vi "Actor Core.vi"(8 "error in":errorcluster, 11 "Nested in":refnum<class "Baratron.lvclass">) -> (0 "error out":errorcluster, 3 "Actor out":refnum<class "Actor.lvclass">)   [LabVIEW 2021, in "Baratron.lvclass"]
doc: "(<B>Filename</B>: Actor Framework.lvlib:Actor.lvclass:Actor Core.vi)\n\nReceives messages to the actor, reacts to them, and initiates any error handling that may shut the actor down.\n\nDescendant classes may override this VI to append parallel tasks for the actor to complete while it handles messages. Overrides use the Call Parent Method node."
uses:
  Baratron.lvclass
  C:/Program Files/National Instruments/LabVIEW 2021/vi.lib/ActorFramework/Actor/Actor.lvclass
  <vilib>/ActorFramework/Actor/Actor.lvclass
  Baratron.lvclass/Baratron.ctl
  <vilib>/ActorFramework/Actor/Actor.lvclass/Actor.ctl
  <vilib>/ActorFramework/Message Enqueuer/Message Enqueuer.lvclass/Message Enqueuer.ctl
  <vilib>/ActorFramework/Message Enqueuer/Init from Existing Queue.vi
  <vilib>/ActorFramework/Message Enqueuer/Enqueue.vi
  <vilib>/ActorFramework/Stop Msg/Stop Msg.lvclass
  C:/Program Files/National Instruments/LabVIEW 2021/vi.lib/ActorFramework/Message/Message.lvclass
  <vilib>/ActorFramework/Message Priority Queue/Priority Enqueue.vi
  <vilib>/MGI/Panel Manager/Panel Actor/Panel Actor/Panel Actor.lvclass
  <vilib>/ActorFramework/Message Enqueuer/Message Enqueuer.lvclass
panel:
  out "Status":string
  out "Baratron Waveform":waveform(dbl)(graph)
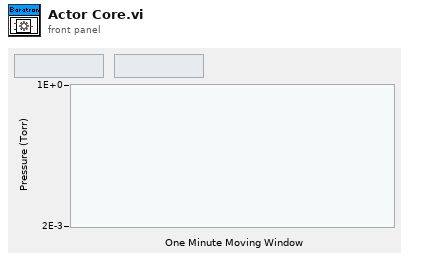
[diagram p1: front panel]
types:
  T1 = cluster{"Stop":refnum<user-event>, "Baratron Waveform":refnum<user-event>, "Status":refnum<user-event>}
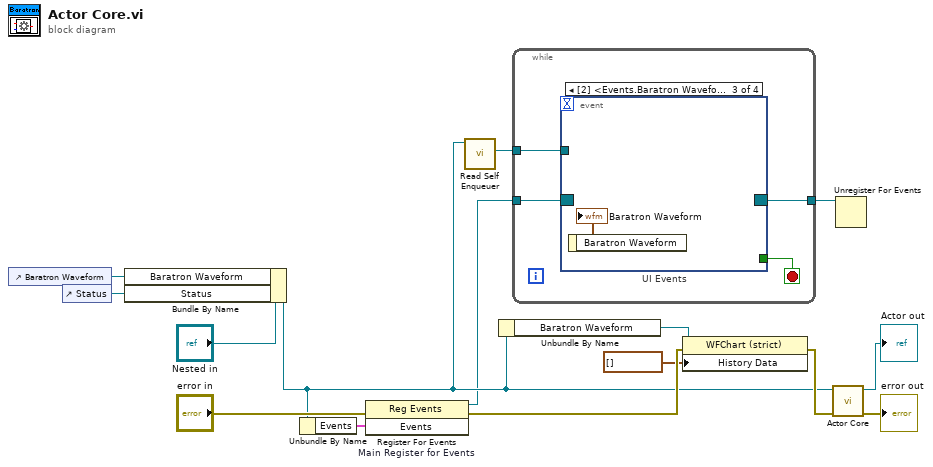
[diagram p0: block diagram]
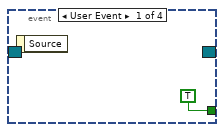
[diagram p2: hidden frame]
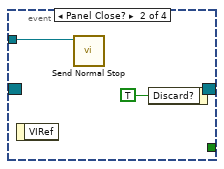
[diagram p3: hidden frame]
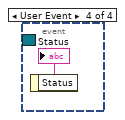
[diagram p4: hidden frame]
diagram:
  n1 = control-ref of="Baratron Waveform"() -> (w1:refnum<vi>)
  n2 = control-ref of="Status"() -> (w11:refnum<vi>)
  n3 = Bundle By Name(cluster="Nested in", "Baratron Waveform"=w1, "Status"=w11) -> (w4:refnum<class "Baratron.lvclass">)
  n4 = Unbundle By Name(w4) -> ("Events"=w13:T1)
  n5 = register-events "Main Register for Events"(error in="error in", w13) -> (reference out=w2:refnum<event-registration>, error out=w6:errorcluster)  [unwired: 1 in]
  n6 = call <vilib>:"Read Self Enqueuer.vi"("Actor"=w4) -> ("Self Enqueuer"=w9:refnum<class "Message Enqueuer.lvclass">)  [unwired: 10 in]
  n7 = Unbundle By Name(w4) -> ("Baratron Waveform"=w7:refnum<vi>)
  n8 = while {
    tunnel: w2 -> [w19]
    tunnel: [w17] -> w12
    tunnel: w9 -> [w16]
    stop <- w18 stop-if-true
    n9 = event "UI Events" shown="[2] <Events.Baratron Waveform>: User Event" {
      selector: w19 -> [_ _ _ _]
      dyn-events: [_ _ _ _] -> w17
      timeout: _ -> [_ _ _ _]
      tunnel: [TRUE _ _ _] -> w18
      tunnel: w16 -> [_ w21 _ _]
      event User Event {
        n10 = event-data() -> ()  [unwired: 1 in, 1 out]
      }
      event Panel Close? {
        n11 = event-data() -> ()  [unwired: 1 in, 1 out]
        n12 = call <vilib>:"Send Normal Stop.vi"("Message Enqueuer"=w21) -> ()  [unwired: 10 in, 1 out]
        n13 = event-data("Discard?"=TRUE) -> ()  [unwired: 1 in, 1 out]
      }
      event User Event {
        n14 = event-data() -> ("Baratron Waveform"=→"Baratron Waveform":waveform(dbl))  [unwired: 1 in]
      }
      event User Event {
        n15 = event-data() -> ("Status"=→"Status":string)  [unwired: 1 in]
      }
    }
  }
  n16 = property class="WFChart (strict)"(reference=w7, error in=w6, "History Data"=waveform(dbl)[] []) -> (error out=w5:errorcluster)  [unwired: 1 out]
  n17 = call-parent "Actor Core.vi"("error in"=w5, "Panel Actor in"=w4) -> ("error out"=→"error out":errorcluster, "Actor out"=→"Actor out":refnum<class "Actor.lvclass">)  [unwired: 8 in]
  n18 = Unregister For Events(event registration refnum=w12) -> ()  [unwired: 1 in, 1 out]
